vi "Bin Devices into Groups.vi"(8 "error in (no error)":errorcluster, 10 "DeviceID Array":T1[](array[typedef]), 11 "Startup Optimization in":refnum<class "Startup Optimization.lvclass">) -> (0 "error out":errorcluster, 3 "Startup Optimization out":refnum<class "Startup Optimization.lvclass">, 4 "Number of PCCs":i16)   [LabVIEW 2018, in "Startup Optimization Actor.lvlib" / "Startup Optimization.lvclass"]
uses:
  Startup Optimization.lvclass
  <vilib>/ORNL/CSEISMIC DDS/CSEISMIC DDS Base/Data Types/Controls/DeviceID.ctl
  Startup Optimization.lvclass/Startup Optimization.ctl
  <vilib>/ORNL/CSEISMIC DDS/CSEISMIC DDS Base/CSEISMIC DDS.lvclass
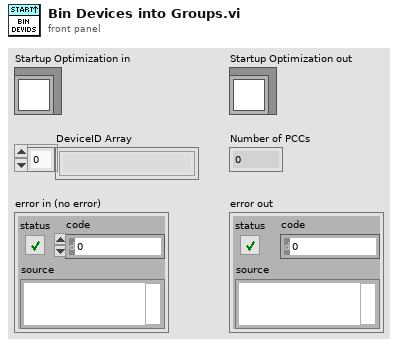
[diagram p1: front panel]
types:
  T1 = typedef "CSEISMIC DDS.lvlib/CSEISMIC DDS.lvclass/DeviceID.ctl" = string
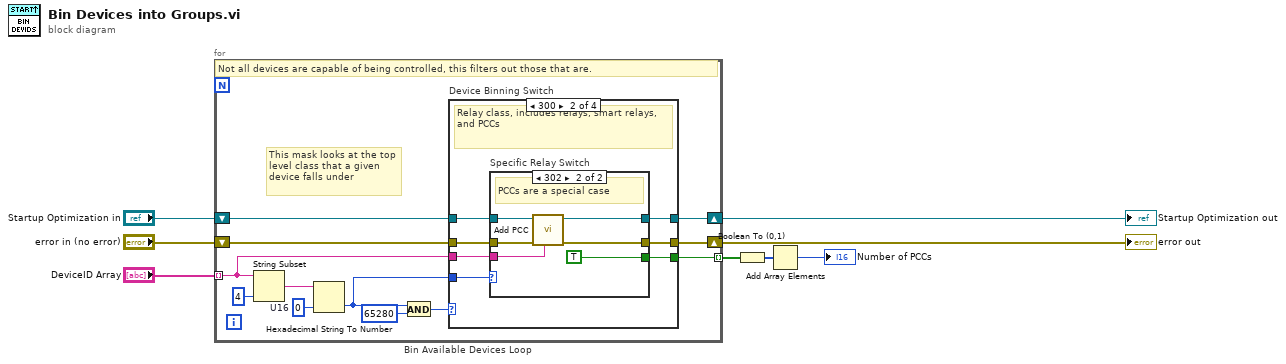
[diagram p0: block diagram]
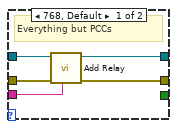
[diagram p3: hidden frame]
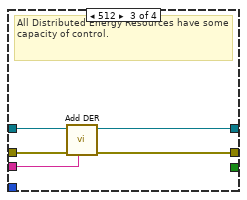
[diagram p4: hidden frame]
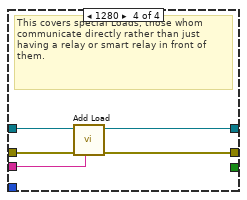
[diagram p5: hidden frame]
diagram:
  n1 = for "Bin Available Devices Loop" {
    tunnel: "DeviceID Array" -> [w18] mode=indexing
    shift-right: [w17] -> w4
    shift-left: "Startup Optimization in" -> [w19]
    tunnel: [w16] -> w1 mode=indexing
    shift-right: [w9] -> w8
    shift-left: "error in (no error)" -> [w10]
    w14 = u16 0  # U16
    # "This mask looks at the top level class that a given device falls under"
    # "Not all devices are capable of being controlled, this filters out those that are."
    n2 = String Subset(string=w18, length (rest)=4 ("length (rest)")) -> (substring=w15:T1)  [unwired: 1 in]
    n3 = Hexadecimal String To Number(string=w15, default (0uL)=w14) -> (number=w11:u16)  [unwired: 1 in, 1 out]
    n4 = And(x=w11, y=u16 65280) -> (x .and. y?=w13:u16)
    n5 = case "Device Binning Switch" shown="300" w13 {
      tunnel: w19 -> [w22 w28 w45 w50]
      tunnel: w18 -> [_ w29 w43 w48]
      tunnel: [w22 w27 w44 w49] -> w17
      tunnel: [_ w25 _ _] -> w16
      tunnel: w11 -> [_ w26 _ _]
      tunnel: w10 -> [w21 w24 w42 w47]
      tunnel: [w21 w23 w41 w46] -> w9
      frame Default {
        # "All devices that are not controled"
      }
      frame 768 {
        # "Relay class, includes relays, smart relays, and PCCs"
        n6 = case "Specific Relay Switch" shown="302" w26 {
          tunnel: w29 -> [w32 w37]
          tunnel: w28 -> [w34 w39]
          tunnel: [w33 w38] -> w27
          tunnel: [_ TRUE] -> w25
          tunnel: w24 -> [w31 w36]
          tunnel: [w30 w35] -> w23
          frame 768, Default {
            # "Everything but PCCs"
            n7 = call "Add Relay.vi"("DeviceID"=w32, "error in"=w31, "Startup Optimization in"=w34) -> ("error out"=w30:errorcluster, "Startup Optimization out"=w33:refnum<class "Startup Optimization.lvclass">)  [unwired: 7 in]
          }
          frame 770 {
            # "PCCs are a special case"
            n8 = call "Add PCC.vi"("DeviceID"=w37, "error in"=w36, "Startup Optimization in"=w39) -> ("error out"=w35:errorcluster, "Startup Optimization out"=w38:refnum<class "Startup Optimization.lvclass">)  [unwired: 7 in]
          }
        }
      }
      frame 512 {
        # "All Distributed Energy Resources have some capacity of control."
        n9 = call "Add DER.vi"("DeviceID"=w43, "error in"=w42, "Startup Optimization in"=w45) -> ("error out"=w41:errorcluster, "Startup Optimization out"=w44:refnum<class "Startup Optimization.lvclass">)  [unwired: 7 in]
      }
      frame 1280 {
        # "This covers special Loads, those whom communicate directly rather than just having a relay or smart relay in front of them."
        n10 = call "Add Load.vi"("DeviceID"=w48, "error in"=w47, "Startup Optimization in"=w50) -> ("error out"=w46:errorcluster, "Startup Optimization out"=w49:refnum<class "Startup Optimization.lvclass">)  [unwired: 7 in]
      }
    }
  }
  "error out" <- w8
  "Startup Optimization out" <- w4
  n11 = Boolean To (0,1)(Boolean=w1) -> (0, 1=w2:i16[])
  n12 = Add Array Elements(numeric array=w2) -> (sum=→"Number of PCCs":i16)
